vi "Pickering 40-295 Driver.vi"(9 "Device Inputs FIFO":refnum<k33>, 10 "Device Outputs FIFO":refnum<k33>, 11 "Device Reference":T1 format="%.0x") -> ()   [LabVIEW 2014, in "Pickering 40-295.lvlib"]
uses:
  Pickering 40-295.lvlib
  <vilib>/NI Veristand/Custom Device API/Custom Device Item Ref.ctl
  <vilib>/NI Veristand/Custom Device API/Custom Device Channel Type.ctl
  <vilib>/NI Veristand/Custom Device API/Get Item Property (String).vi
  <vilib>/NI Veristand/Custom Device API/Custom Device API.lvlib
panel:
  in  "Initialization Status Notifier":refnum<notifier>
  in  "Status Notifier":refnum<notifier>
  # "Custom Device Template\nv1.0"
  # "Use this template as a starting point for creating a custom device code module. The input controls shown here are specially named controls that the system will use to provide the device loop with data. The controls are not required for the device loop to run. For instance, if the device doesn't produce any output data, then you don't need the Device Outputs FIFO control. If you do use these controls, however, they need to have these exact names to be functional."
  # "The status queue element is used to signalize the RT engine that the last state of the custom device."
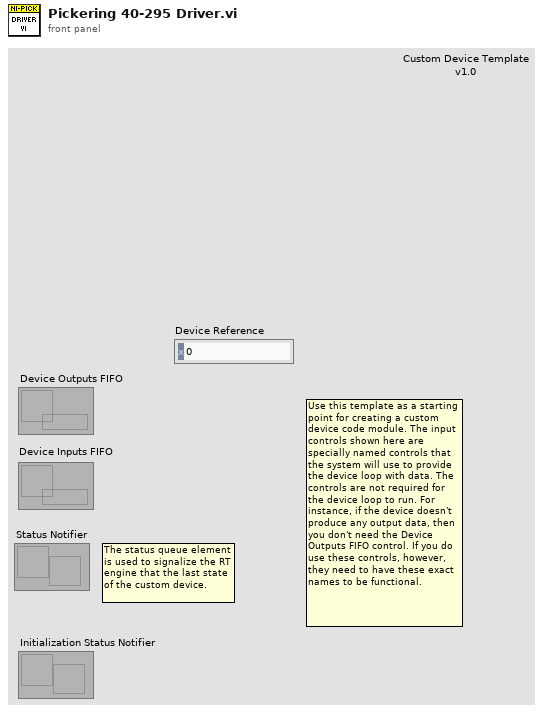
[diagram p1: front panel]
types:
  T1 = typedef "Custom Device API.lvlib/Custom Device Item Ref.ctl" = u64
  T2 = typedef "Custom Device API.lvlib/Custom Device Channel Type.ctl" = enum16{"Input", "Output"}
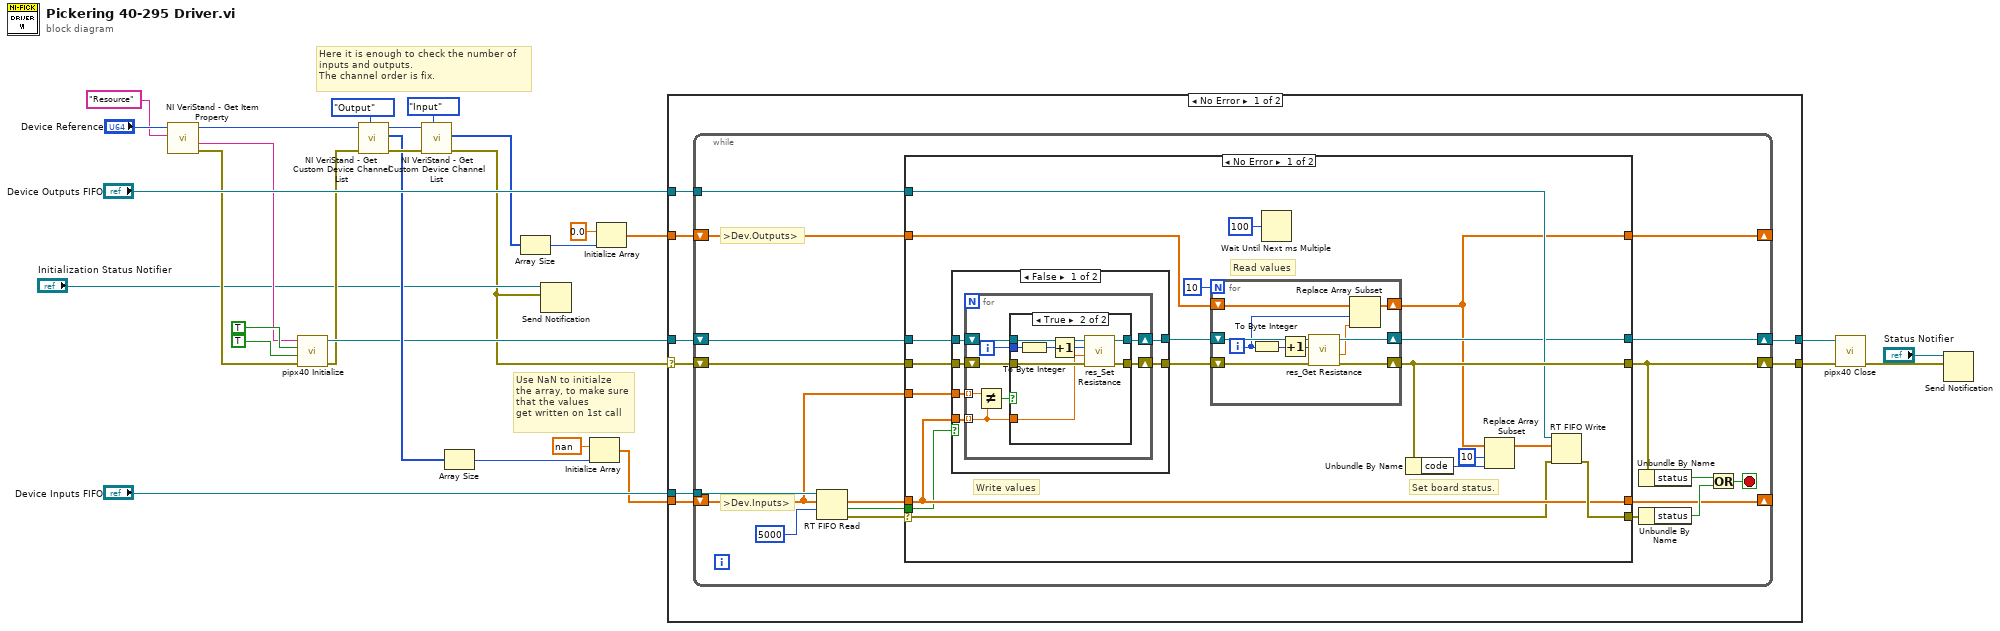
[diagram p0: block diagram]
diagram:
  # "Here it is enough to check the number of\ninputs and outputs.\nThe channel order is fix."
  # "Use NaN to initialze\nthe array, to make sure\nthat the values\nget written on 1st call"
  n1 = call-poly <vilib>:"NI VeriStand - Get Item Property.vi"("Property Name"="Resource", "Item Ref in"="Device Reference") -> ("error out"=w11:errorcluster, "Value"=w3:string, "Item Ref out"=w12:T1)  [unwired: 2 in, 5 out]
  n2 = call "pipx40 Initialize.vi"("error in (no error)"=w11, "reset device"=TRUE, "id query"=TRUE, "resource name"=w3) -> ("error out"=w9:errorcluster, "instrument handle out"=w10:refnum<visa-resource-name>)  [unwired: 6 out]
  n3 = call <vilib>:"NI VeriStand - Get Custom Device Channel List.vi"("Channel Type"=Custom_Device_Channel_Type."Output", "error in (no error)"=w9, "Device Ref in"=w12) -> ("error out"=w21:errorcluster, "Specified Channel Ref List"=w18:T1[], "Device Ref out"=w22:T1)  [unwired: 6 out]
  n4 = call <vilib>:"NI VeriStand - Get Custom Device Channel List.vi"("Channel Type"=Custom_Device_Channel_Type."Input", "error in (no error)"=w21, "Device Ref in"=w22) -> ("error out"=w1:errorcluster, "Specified Channel Ref List"=w16:T1[])  [unwired: 7 out]
  n5 = Array Size(array=w18) -> (size(s)=w17:i32)
  n6 = Array Size(array=w16) -> (size(s)=w8:i32)
  n7 = Send Notification(notification=w1, notifier="Initialization Status Notifier") -> ()  [unwired: 1 in, 2 out]
  n8 = Initialize Array(nan ("element"), w17) -> (w24:dbl[])
  n9 = Initialize Array(0.0 ("element"), w8) -> (w25:dbl[])
  n10 = case shown="No Error" w1 {
    selector: w1 -> [w30 w117]
    tunnel: "Device Outputs FIFO" -> [w37 _]
    tunnel: "Device Inputs FIFO" -> [w36 _]
    tunnel: w25 -> [w35 _]
    tunnel: w24 -> [w34 _]
    tunnel: w10 -> [w33 w116]
    tunnel: [w32 w116] -> w7
    tunnel: [w31 w117] -> w6
    frame No Error {
      n11 = while {
        shift-right: [w42] -> _
        shift-left: w34 -> [w51]
        shift-right: [w40] -> w31
        shift-left: w30 -> [w41]
        shift-right: [w47] -> _
        shift-left: w35 -> [w48]
        tunnel: w37 -> [w55]
        tunnel: w36 -> [w54]
        shift-right: [w45] -> w32
        shift-left: w33 -> [w49]
        stop <- w39 stop-if-true
        # ">Dev.Outputs>"
        # ">Dev.Inputs>"
        n12 = RT FIFO Read(0:w54, 1:w51, 2:5000 ("timeout in ms (0)")) -> (9:w52:dbl[], 10:w50:bool, 11:w43:errorcluster)  [unwired: 1 in, 2 out]
        n13 = case shown="No Error" w43 {
          selector: w43 -> [w61 w115]
          tunnel: w55 -> [w73 _]
          tunnel: w52 -> [w65 w113]
          tunnel: w51 -> [w72 _]
          tunnel: w50 -> [w56 _]
          tunnel: w49 -> [w71 w112]
          tunnel: w48 -> [w68 w114]
          tunnel: [w60 w114] -> w47
          tunnel: [w67 w112] -> w45
          tunnel: [w66 w115] -> w44
          tunnel: [w74 w111] -> w40
          tunnel: [w65 w113] -> w42
          tunnel: w41 -> [w62 w111]
          frame No Error {
            # "Set board status."
            # "Read values"
            # "Write values"
            n14 = case shown="False" w56 {
              tunnel: w65 -> [w90 _]
              tunnel: w72 -> [w89 _]
              tunnel: w71 -> [w88 w110]
              tunnel: [w87 w110] -> w70
              tunnel: w62 -> [w86 w109]
              tunnel: [w85 w109] -> w69
              frame False {
                n15 = for {
                  tunnel: w90 -> [w95] mode=indexing
                  tunnel: w89 -> [w97] mode=indexing
                  shift-right: [w93] -> w87
                  shift-left: w88 -> [w96]
                  shift-right: [w91] -> w85
                  shift-left: w86 -> [w92]
                  i -> [w94]
                  n16 = Not Equal?(x=w97, y=w95) -> (x != y?=w98:bool)
                  n17 = case shown="True" w98 {
                    tunnel: w96 -> [w100 w108]
                    tunnel: [w100 w107] -> w93
                    tunnel: w95 -> [_ w101]
                    tunnel: w94 -> [_ w105]
                    tunnel: w92 -> [w99 w103]
                    tunnel: [w99 w102] -> w91
                    frame False {
                    }
                    frame True {
                      n18 = To Byte Integer(number=w105) -> (8bit integer=w104:i8)
                      n19 = Increment(x=w104) -> (x+1=w106:i8)
                      n20 = call "res_Set Resistance.vi"("error in (no error)"=w103, "Resistance (0-65535 Ohms)"=w101, "Channel (1-10)"=w106, "instrument handle"=w108) -> ("error out"=w102:errorcluster, "instrument handle out"=w107:refnum<visa-resource-name>)  [unwired: 6 out]
                    }
                  }
                }
              }
              frame True {
              }
            }
            n21 = for {
              N: 10 -> [_]
              shift-right: [w75] -> w60
              shift-left: w68 -> [w78]
              shift-right: [w83] -> w67
              shift-left: w70 -> [w84]
              shift-right: [w81] -> w74
              shift-left: w69 -> [w82]
              i -> [w76]
              n22 = To Byte Integer(number=w76) -> (8bit integer=w80:i8)
              n23 = Increment(x=w80) -> (x+1=w79:i8)
              n24 = call "res_Get Resistance.vi"("error in (no error)"=w82, "Channel (1-10)"=w79, "instrument handle"=w84) -> ("error out"=w81:errorcluster, "Actual Resistance"=w77:dbl, "instrument handle out"=w83:refnum<visa-resource-name>)  [unwired: 6 out]
              n25 = Replace Array Subset(array=w78, new element=w77, index=w76) -> (w75:dbl[])
            }
            n26 = Wait Until Next ms Multiple(millisecond multiple=u32 100) -> ()  [unwired: 1 out]
            n27 = Unbundle By Name(w74) -> ("code"=w58:i32)
            n28 = Replace Array Subset(array=w60, new element=w58, index=10) -> (w57:dbl[])
            n29 = RT FIFO Write(0:w73, 1:w57, 3:w61) -> (11:w66:errorcluster)  [unwired: 1 in, 4 out]
          }
          frame Error {
          }
        }
        n30 = Unbundle By Name(w40) -> ("status"=w38:bool)
        n31 = Unbundle By Name(w44) -> ("status"=w46:bool)
        n32 = Or(x=w38, y=w46) -> (x .or. y?=w39:bool)
      }
    }
    frame Error {
    }
  }
  n33 = call "pipx40 Close.vi"("error in (no error)"=w6, "instrument handle"=w7) -> ("error out"=w5:errorcluster)  [unwired: 9 out]
  n34 = Send Notification(notification=w5, notifier="Status Notifier") -> ()  [unwired: 1 in, 2 out]
